vi "createChannel.vi"(8 "error in (no error)":errorcluster, 11 "AnalogOutput in":refnum<class "AnalogOutput.lvclass">) -> (0 "error out":errorcluster, 3 "AnalogOutput out":refnum<class "AnalogOutput.lvclass">)   [LabVIEW 2009, in "Hardware.lvlib" / "Channels.lvlib" / "AnalogOutput.lvclass"]
doc: "Abstract Method.\n\nCreates an analog output channel by reserving hardware resources needed by the output. This vi sets a name for the channel, and via its implementation classes (such as niDAQmxAO etc) reserves the physical channel on the output device."
uses:
  AnalogOutput.lvclass
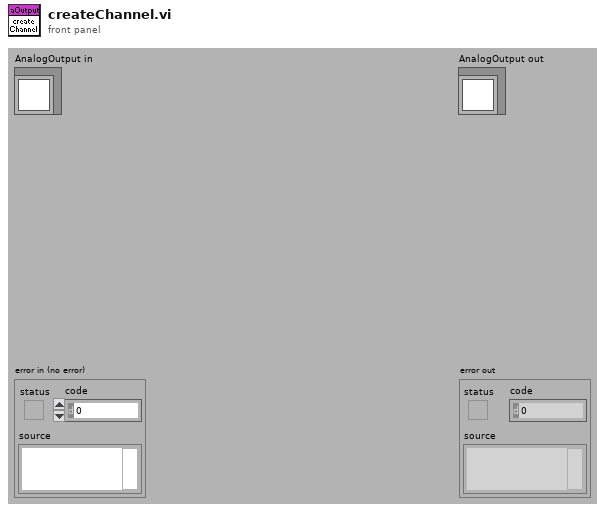
[diagram p1: front panel]
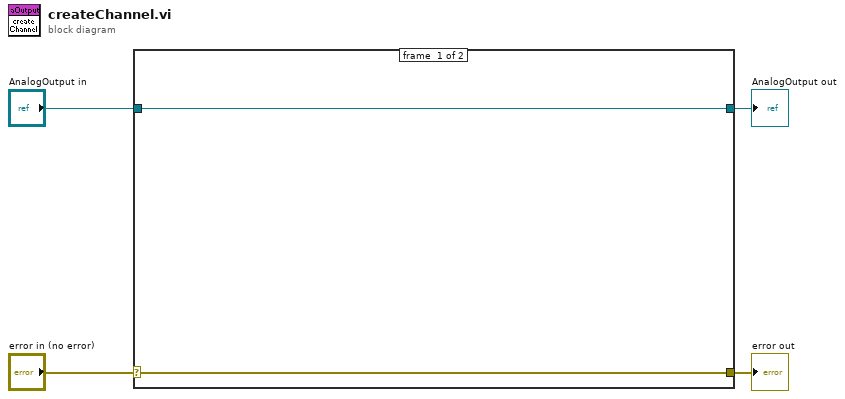
[diagram p0: block diagram]
diagram:
  n1 = case shown="No Error" "error in (no error)" {
    selector: "error in (no error)" -> [w6 w8]
    tunnel: [w6 w8] -> w3
    tunnel: [w5 w7] -> w1
    tunnel: "AnalogOutput in" -> [w5 w7]
    frame #0 {
    }
    frame #1 {
    }
  }
  "error out" <- w3
  "AnalogOutput out" <- w1
